vi "Write UI References.vi"(8 "error in (no error)":errorcluster, 10 "UI References":T1, 11 "Results in":refnum<class "Results.lvclass">) -> (0 "error out":errorcluster, 3 "Results out":refnum<class "Results.lvclass">)   [LabVIEW 2016, in "Result Actor.lvlib" / "Results.lvclass"]
uses:
  Results.lvclass
  UI References.ctl
  Results.lvclass/Results.ctl
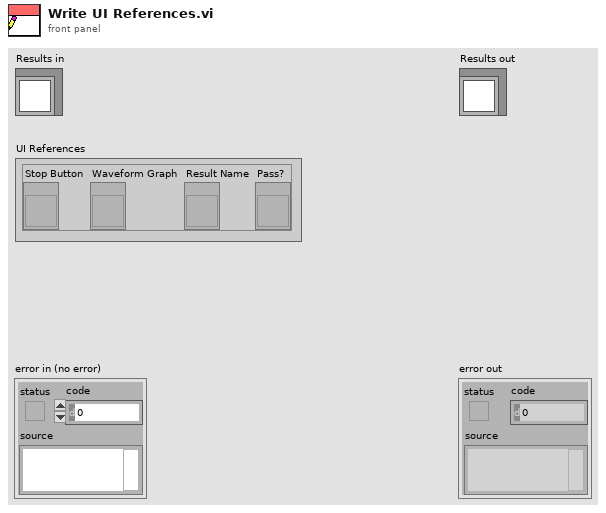
[diagram p1: front panel]
types:
  T1 = typedef "Result Actor.lvlib/Results.lvclass/UI References.ctl" = cluster{"Stop Button":refnum<vi>, "Waveform Graph":refnum<vi>, "Result Name":refnum<vi>, "Pass?":refnum<vi>}
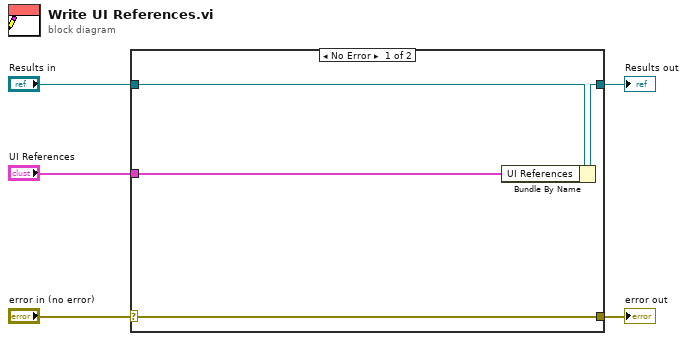
[diagram p0: block diagram]
diagram:
  n1 = case shown="No Error" "error in (no error)" {
    selector: "error in (no error)" -> [w9 w10]
    tunnel: [w9 w10] -> w4
    tunnel: [w7 w11] -> w2
    tunnel: "Results in" -> [w8 w11]
    tunnel: "UI References" -> [w6 _]
    frame No Error {
      n2 = Bundle By Name(cluster=w8, "UI References"=w6) -> (w7:refnum<class "Results.lvclass">)
    }
    frame Error {
    }
  }
  "error out" <- w4
  "Results out" <- w2
